vi "MH_Count_Records.vi"(8 "error in (no error)":errorcluster caption="entrée d'erreur (pas d'erreur)", 11 "RecBuffer":u32[](array[numeric])) -> (0 "error out":errorcluster caption="sortie d'erreur", 3 "Photon Counts":u32)   [LabVIEW 2019]
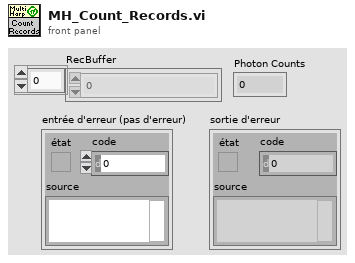
[diagram p1: front panel]
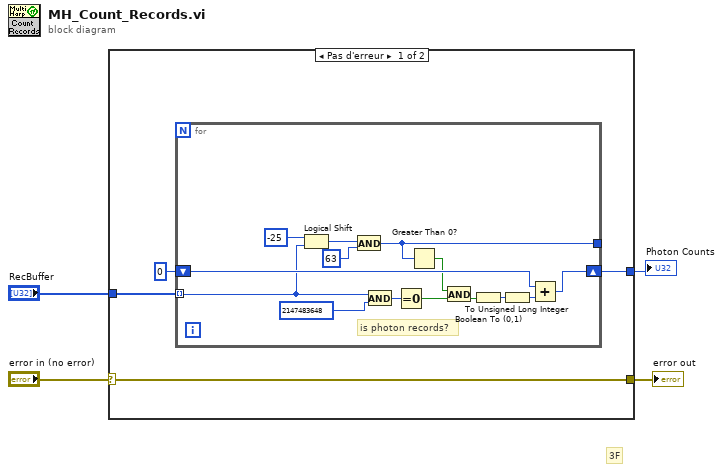
[diagram p0: block diagram]
diagram:
  # "3F"
  n1 = case shown="Pas d'erreur" "error in (no error)" {
    selector: "error in (no error)" -> [w5 w23]
    tunnel: [w5 w23] -> w1
    tunnel: "RecBuffer" -> [w8 _]
    tunnel: [w6 _] -> w2
    frame No Error {
      n2 = for {
        tunnel: w8 -> [w14] mode=indexing
        shift-right: [w18] -> w6
        shift-left: u32 0 -> [w17]
        tunnel: [w9] -> _
        # "is photon records?"
        n3 = Logical Shift(y=i16 -25, x=w14) -> (x << y=w13:u32)
        n4 = And(x=w13, y=u32 63) -> (x .and. y?=w9:u32)
        n5 = And(x=w14, y=u32 2147483648 ("x")) -> (x .and. y?=w21:u32)
        n6 = Equal To 0?(x=w21) -> (x = 0?=w20:bool)
        n7 = Greater Than 0?(x=w9) -> (x > 0?=w10:bool)
        n8 = And(x=w10, y=w20) -> (x .and. y?=w11:bool)
        n9 = Boolean To (0,1)(Boolean=w11) -> (0, 1=w19:i16)
        n10 = To Unsigned Long Integer(number=w19) -> (unsigned 32bit integer=w16:u32)
        n11 = Add(x=w17, y=w16) -> (x+y=w18:u32)
      }
    }
    frame Error {
    }
  }
  "error out" <- w1
  "Photon Counts" <- w2
